vi "Subtract Float SCTL 40 MHz Latency 1.vi"(2 "y":sgl, 3 "x":sgl) -> (0 "ready":bool=TRUE, 1 "x[k-1]-y[k-1]":sgl)   [LabVIEW 2017]
uses:
  <vilib>/rvi/XilinxIP/XIPIN_XNode/niFpgaXIPIN.xnode
  <vilib>/rvi/IPIntegrationNode/IPINode_Xnode/niFpgaIPINode.xnode
  <vilib>/rvi/IPIntegrationNode/IPINode_Typedef/niFpgaIPINodeSupportedFamilies.ctl
  <vilib>/rvi/IPIntegrationNode/IPINode_Utilities/niFpgaIPINodeSimCore.vi
  Subtract SCTL L1/Subtract_SCTL_L1_C3ADE5BE76064AA39E7EE6565DE88692.dll
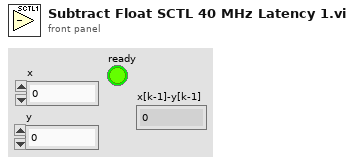
[diagram p1: front panel]
types:
  T1 = typedef "niFpgaIPINodeSupportedFamilies.ctl" = cluster{"unlimited?":bool, "supported targets":string[]}
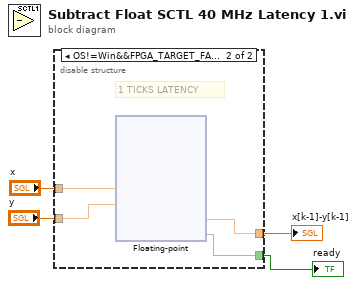
[diagram p0: block diagram]
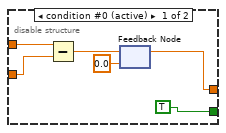
[diagram p2: hidden frame]
diagram:
  n1 = disable-structure shown="OS!=Win&&FPGA_TARGET_FAMILY==SPARTAN6" {
    disable-tunnel: "x" -> [w10 w14]
    disable-tunnel: [w7 w12] -> w2
    disable-tunnel: "y" -> [w9 w13]
    disable-tunnel: [TRUE w11] -> w1
    frame condition #0 (active) {
      n2 = Subtract(x=w10, y=w9) -> (x-y=w8:sgl)
      n3 = feedback-in #1(w8) -> ()
      n4 = feedback #1(sgl 0.0) -> (w7:sgl)
    }
    frame condition #1 {
      # "1 TICKS LATENCY"
      n5 = xnode ("Floating-point")("a"=w14, "b"=w13) -> ("result"=w12:sgl, "rdy"=w11:bool)  [unwired: 2 in]
    }
  }
  "x[k-1]-y[k-1]" <- w2
  "ready" <- w1
